vi "Verify MyAnd Parameterized.vi"(8 "error in":errorcluster) -> (0 "error out":errorcluster)   [LabVIEW 2020]
uses:
  <vilib>/SAS/Approval Tests/Extensions/Caraya.Extension/lib_Caraya.Extension.lvlib
  <vilib>/addons/_JKI Toolkits/Caraya/classes/Test/Test.lvclass
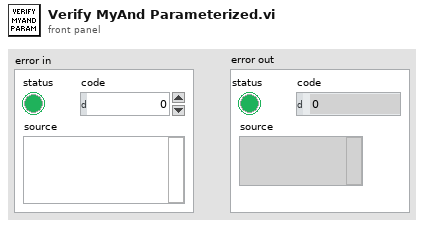
[diagram p1: front panel]
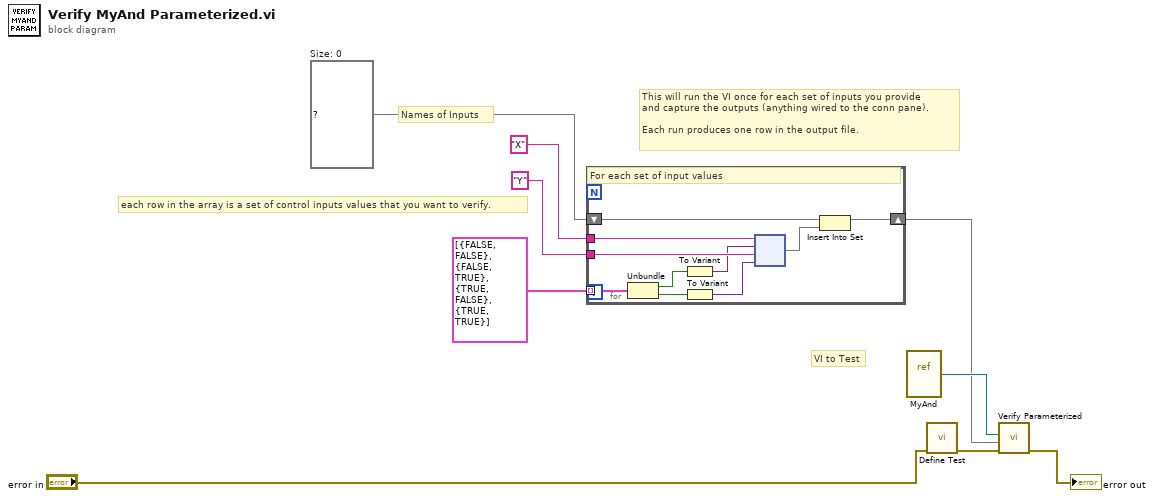
[diagram p0: block diagram]
diagram:
  w6 = set{map{string, variant}} {}  # Size: 0
  # "This will run the VI once for each set of inputs you provide\nand capture the outputs (anything wired to the conn pane).\n\nEach run produces one row in the output file."
  # "VI to Test"
  # "each row in the array is a set of control inputs values that you want to verify."
  # "Names of Inputs"
  n1 = for {
    tunnel: "X" -> [w19]
    tunnel: cluster{bool, bool}[] [{FALSE, FALSE}, {FALSE, TRUE}, {TRUE, FALSE}, {TRUE, TRUE}] -> [w17] mode=indexing
    tunnel: "Y" -> [w18]
    shift-right: [w11] -> w1
    shift-left: w6 -> [w10]
    # "For each set of input values"
    n2 = Unbundle(w17) -> (w16:bool, w15:bool)
    n3 = To Variant(anything=w16) -> (Variant=w13:variant)
    n4 = To Variant(anything=w15) -> (Variant=w12:variant)
    n5 = node(w19, w13, w18, w12) -> (w14:map{string, variant})
    n6 = Insert Into Set(10:w14, 11:w10) -> (3:w11:set{map{string, variant}})  [unwired: 1 out]
  }
  n7 = vi-ref "MyAnd.vi"() -> (w2:refnum<vi>)
  n8 = call <vilib>:"Define Test.vi"("error in (no error)"="error in") -> ("error out"=w9:errorcluster)  [unwired: 9 in, 1 out]
  n9 = call <vilib>:"Verify Parameterized.vi"("error in"=w9, "ctl label -> value var"=w1, "VI Refnum"=w2) -> ("error out"=→"error out":errorcluster)  [unwired: 7 in, 1 out]
